vi "JPL Encoder PID (SubVI).vi"(4 "refnum name":string, 5 "Encoder Config":T1, 6 "PID Settings":T3, 7 "PID Limits":cluster{"Upper Limit":dbl, "Lower Limit":dbl}) -> (0 "Encoder Status":T2, 3 "output":dbl)   [LabVIEW 2015]
uses:
  <vilib>/functionblocks/Edge Detection/One Shot Rising with Input/One Shot Rising with Input.vi
  <vilib>/addons/control/pid/pid.llb/PID (DBL).vi
  <vilib>/functionblocks/FB Core/FB Core.xnode
  <vilib>/addons/control/pid/NI_PID_pid.lvlib
  <vilib>/functionblocks/NI_FunctionBlock Libraries.lvlib
panel:
  out "Encoder Distance Chart":dbl(graph)
  out "PID Output Chart":dbl(graph)
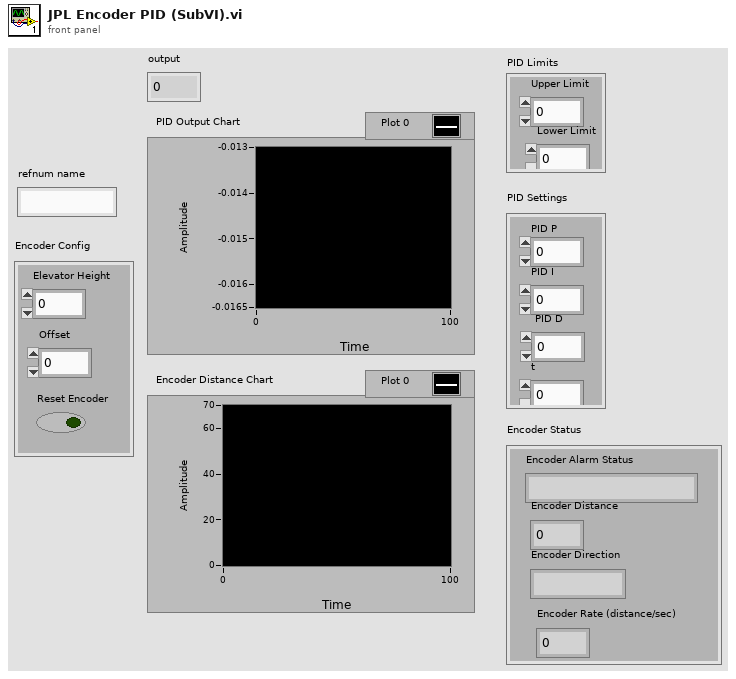
[diagram p1: front panel]
types:
  T1 = cluster{"Elevator Height":dbl, "Offset":dbl, "Reset Encoder":bool}
  T2 = cluster{"Encoder Alarm Status":string, "Encoder Distance":dbl, "Encoder Direction":string, "Encoder Rate (distance/sec)":dbl}
  T3 = cluster{"PID P":dbl, "PID I":dbl, " PID D":dbl, "t":dbl}
  T4 = typedef "WPI_EncoderDevRef.ctl" = cluster{"DevStatus":errorcluster, "EncoderIndex":T5, "CounterIndex":T6, "DistancePerCount":dbl, "Decoding Type":T7}
  T5 = typedef "FPGA_EncoderIdx.ctl" = enum8{"Enc 0", "Enc 1", "Enc 2", "Enc 3", "Enc 4", "Enc 5", "Enc 6", "Enc 7", "Invalid"}
  T6 = typedef "FPGA_CounterCtrSystemIndex.ctl" = enum8{"Ctr 0", "Ctr 1", "Ctr 2", "Ctr 3", "Ctr 4", "Ctr 5", "Ctr 6", "Ctr 7", "Invalid"}
  T7 = typedef "WPI_EncoderType.ctl" = enum16{"1x", "2x", "4x"}
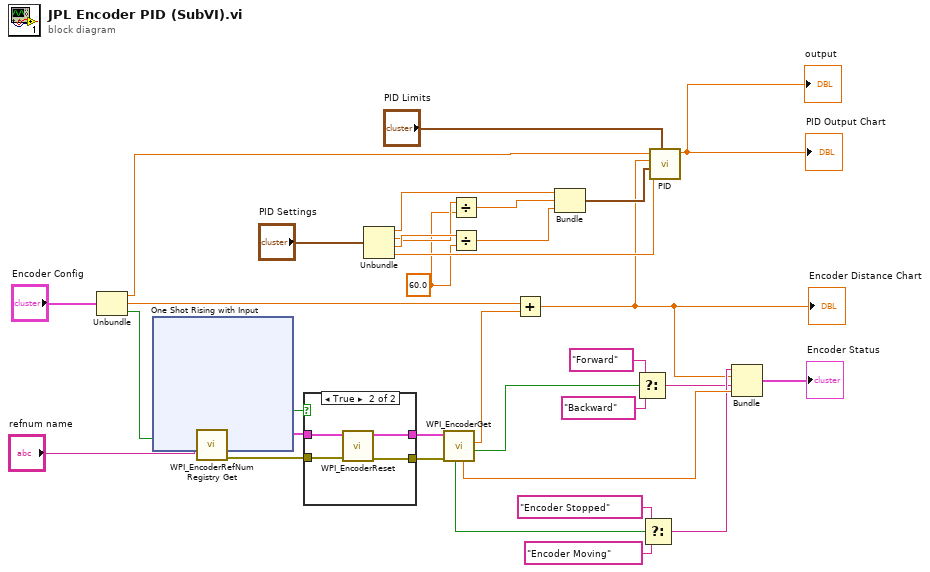
[diagram p0: block diagram]
diagram:
  w1 = 60.0
  n1 = Unbundle("Encoder Config") -> ("Elevator Height"=w7:dbl, "Offset"=w8:dbl, "Reset Encoder"=w9:bool)
  n2 = xnode "One Shot Rising with Input"("input"=w9) -> ("output"=w33:bool)  [unwired: 1 in, 1 out]
  n3 = call <vilib>:"WPI_EncoderRefNum Registry Get.vi"("refnum name"="refnum name") -> ("error out"=w22:errorcluster, "EncoderDevRef"=w21:T4)  [unwired: 9 in]
  n4 = case shown="True" w33 {
    tunnel: w21 -> [w35 w36]
    tunnel: [w35 w39] -> w24
    tunnel: w22 -> [w34 w38]
    tunnel: [w34 w37] -> w31
    frame False {
    }
    frame True {
      n5 = call <vilib>:"WPI_EncoderReset.vi"("error in (no error)"=w38, "EncoderDevRef"=w36) -> ("error out"=w37:errorcluster, "EncoderDevRef"=w39:T4)  [unwired: 8 out]
    }
  }
  n6 = Unbundle("PID Settings") -> ("PID P"=w3:dbl, "PID I"=w5:dbl, "PID D"=w6:dbl, "t"=w17:dbl)
  n7 = call <vilib>:"WPI_EncoderGet.vi"("error in (no error)"=w31, "EncoderDevRef"=w24) -> ("Direction"=w25:bool, "Distance"=w32:dbl, "Rate"=w14:dbl, "Stopped"=w26:bool)  [unwired: 6 out]
  n8 = Divide(x=w5, y=w1) -> (x/y=w2:dbl)
  n9 = Divide(x=w6, y=w1) -> (x/y=w4:dbl)
  n10 = Add(x=w8, y=w32) -> (x+y=w11:dbl)
  "Encoder Distance Chart" <- w11
  n11 = Bundle("PID P"=w3, w2, w4) -> (w16:cluster{"PID P":dbl, dbl, dbl})  [unwired: 1 in]
  n12 = Select(t="Forward", s=w25, f="Backward") -> (s? t:f=w12:string)
  n13 = Select(t="Encoder Stopped", s=w26, f="Encoder Moving") -> (s? t:f=w13:string)
  n14 = call-poly <vilib>:"PID.vi"("output range"="PID Limits", "dt (s)"=w17, "PID gains"=w16, "process variable"=w11, "setpoint"=w7) -> ("output"=→"PID Output Chart" →"output":dbl)  [unwired: 5 in, 1 out]
  n15 = Bundle("f"=w13, w11, "f"=w12, "Rate"=w14) -> (→"Encoder Status":cluster{"f":string, dbl, "f":string, "Rate":dbl})  [unwired: 1 in]
